vi "New motor Control.vi"(0 "Encoder 0":dbl, 1 "Encoder 1":dbl, 2 "Encoder 2":dbl, 3 "xTargetSpeed":dbl, 4 "yTargetSpeed":dbl, 5 "wTargetSpeed":dbl) -> (14 "M2":dbl format="%.2f", 15 "M0":dbl format="%.2f", 16 "M1":dbl format="%.2f")   [LabVIEW 2018]
uses:
  <vilib>/addons/control/pid/pid.llb/PID (DBL).vi
  <vilib>/addons/control/pid/NI_PID_pid.lvlib
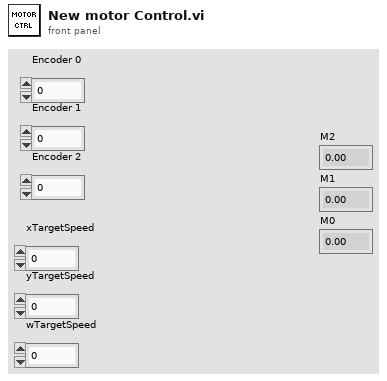
[diagram p1: front panel]
types:
  T1 = cluster{"Encoder 0":dbl, "Encoder 1":dbl, "Encoder 2":dbl}
  T2 = cluster{"proportional gain (Kc)":dbl, "integral time (Ti, min)":dbl, "derivative time (Td, min)":dbl}
  T3 = cluster{"xSpeed":dbl, "ySpeed":dbl, "wSpeed":dbl}
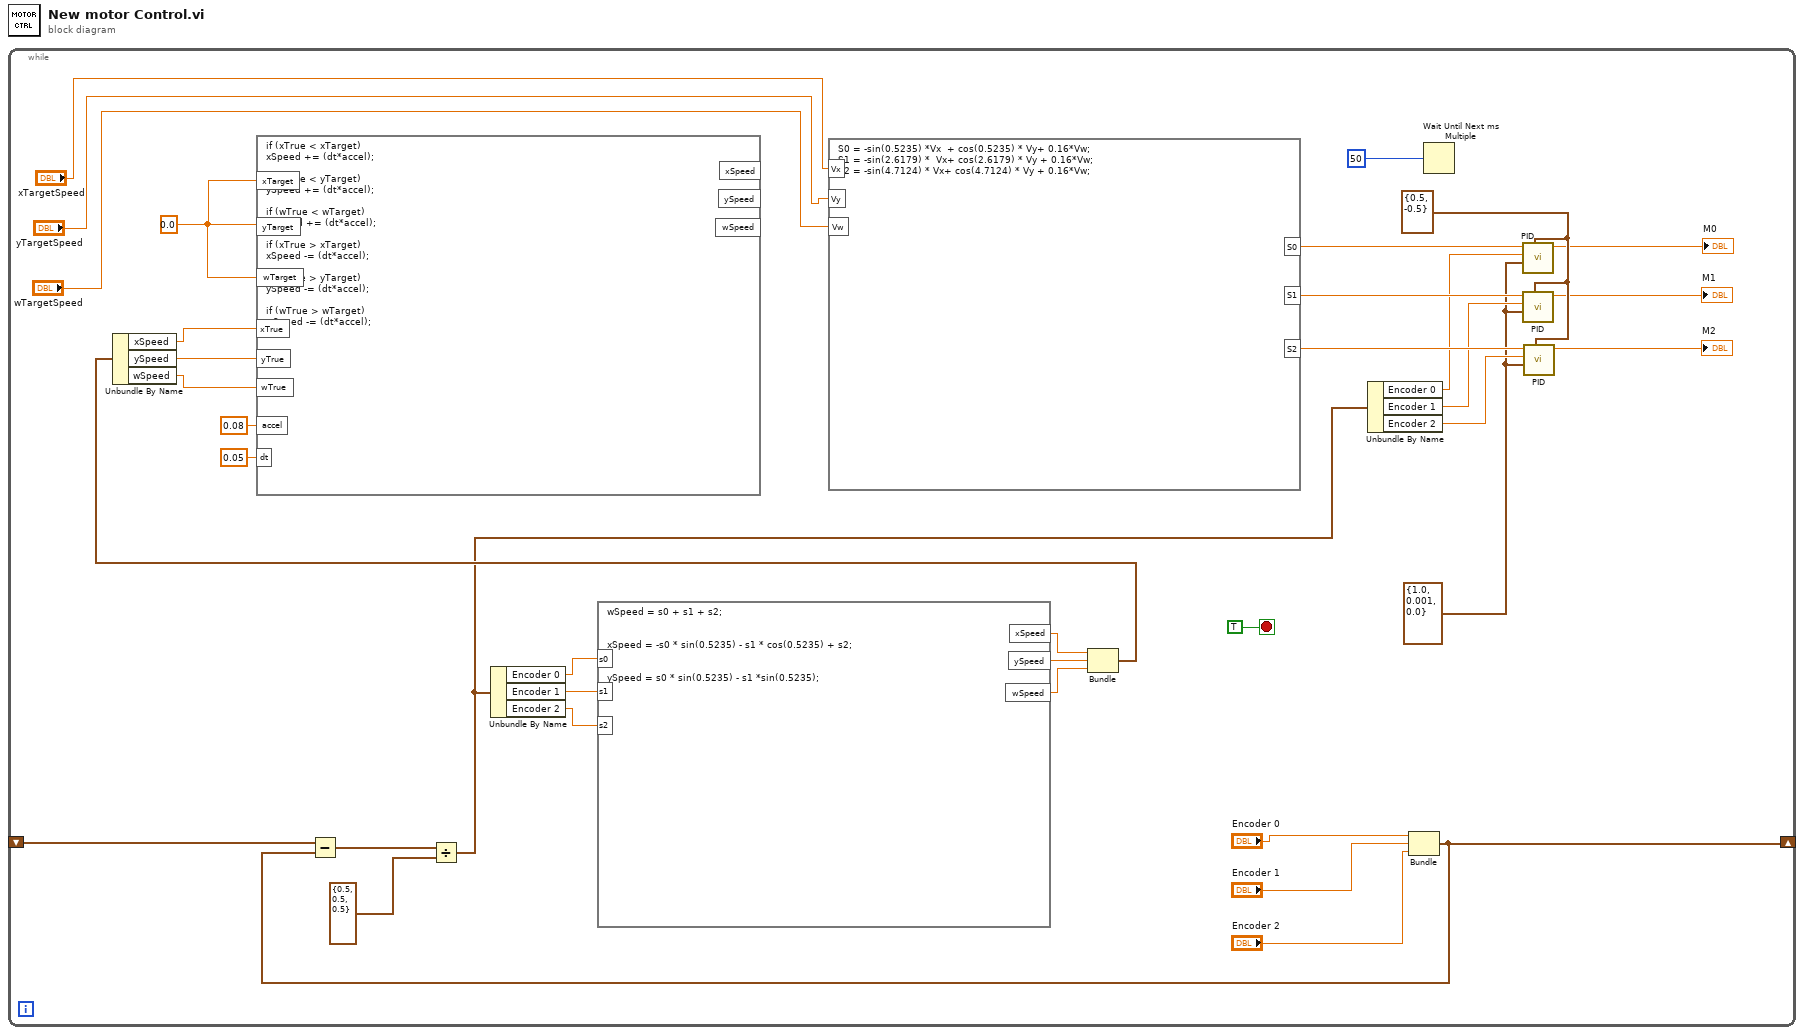
[diagram p0: block diagram]
diagram:
  n1 = while {
    shift-right: [w32] -> _
    shift-left: _ -> [w33]
    stop <- TRUE stop-if-true
    w1 = 0.0
    w11 = cluster{"output high":dbl, "output low":dbl} {"output high"=0.5, "output low"=-0.5} ("output range")
    w12 = T2 {"proportional gain (Kc)"=1.0, "integral time (Ti, min)"=0.001, "derivative time (Td, min)"=0.0} ("PID gains")
    n2 = formula code="S0 = -sin(0.5235) *Vx  + cos(0.5235) * Vy+ 0.16*Vw;\nS1 = -sin(2.6179) *  Vx+ cos(2.6179) * Vy + 0.16*Vw;\nS2 = -sin(4.7124) * Vx+ cos(4.7124) * Vy + 0.16*Vw;"("Vx"="xTargetSpeed", "Vy"="yTargetSpeed", "Vw"="wTargetSpeed") -> ("S0"=w19:dbl, "S1"=w18:dbl, "S2"=w17:dbl)
    n3 = Bundle("Encoder 0"="Encoder 0", "Encoder 1"="Encoder 1", "Encoder 2"="Encoder 2") -> (w32:T1)  [unwired: 1 in]
    n4 = Subtract(x=w33, y=w32) -> (x-y=w31:T1)
    n5 = Divide(x=w31, y=T1 {"Encoder 0"=0.5, "Encoder 1"=0.5, "Encoder 2"=0.5}) -> (x/y=w16:T1)
    n6 = Unbundle By Name(w16) -> ("Encoder 0"=w28:dbl, "Encoder 1"=w29:dbl, "Encoder 2"=w27:dbl)
    n7 = formula code="wSpeed = s0 + s1 + s2;\n\n\nxSpeed = -s0 * sin(0.5235) - s1 * cos(0.5235) + s2;\n\n\nySpeed = s0 * sin(0.5235) - s1 *sin(0.5235);"("s0"=w28, "s1"=w29, "s2"=w27) -> ("xSpeed"=w25:dbl, "ySpeed"=w26:dbl, "wSpeed"=w24:dbl)
    n8 = Bundle("xSpeed"=w25, "ySpeed"=w26, "wSpeed"=w24) -> (w23:T3)  [unwired: 1 in]
    n9 = Unbundle By Name(w23) -> ("xSpeed"=w22:dbl, "ySpeed"=w21:dbl, "wSpeed"=w20:dbl)
    n10 = formula code="if (xTrue < xTarget)\nxSpeed += (dt*accel);\n\nif (yTrue < yTarget)\nySpeed += (dt*accel);\n\nif (wTrue < wTarget)\nwSpeed += (dt*accel);\n\nif (xTrue > xTarget)\nxSpeed -= (dt*accel);\n\nif (yTrue > yTarget)\nySpeed -= (dt*accel);\n\nif (wTrue > wTarget)\nwSpeed -= (dt*accel);"("xTarget"=w1, "yTarget"=w1, "wTarget"=w1, "xTrue"=w22, "yTrue"=w21, "wTrue"=w20, "accel"=0.08 ("input variable"), "dt"=0.05 ("input variable")) -> ()  [unwired: 3 out]
    n11 = Unbundle By Name(w16) -> ("Encoder 0"=w15:dbl, "Encoder 1"=w14:dbl, "Encoder 2"=w13:dbl)
    n12 = Wait Until Next ms Multiple(millisecond multiple=u32 50) -> ()  [unwired: 1 out]
    n13 = call-poly <vilib>:"PID.vi"("output range"=w11, "PID gains"=w12, "process variable"=w15, "setpoint"=w19) -> ("output"=→"M0":dbl)  [unwired: 6 in, 1 out]
    n14 = call-poly <vilib>:"PID.vi"("output range"=w11, "PID gains"=w12, "process variable"=w14, "setpoint"=w18) -> ("output"=→"M1":dbl)  [unwired: 6 in, 1 out]
    n15 = call-poly <vilib>:"PID.vi"("output range"=w11, "PID gains"=w12, "process variable"=w13, "setpoint"=w17) -> ("output"=→"M2":dbl)  [unwired: 6 in, 1 out]
  }
